vi "Add RPC Impl VIs.vi"(8 "error in":errorcluster, 9 "Application reference in":refnum<vi>, 10 "Service Impl class in":refnum<vi>, 11 "RPC Method Parameters":T1[](array[typedef])) -> (0 "error out":errorcluster, 3 "Service Impl class out":refnum<vi>)   [LabVIEW 2019, in "gRPC Template Creation Utility.lvlib"]
uses:
  gRPC Template Creation Utility.lvlib
  TypeDefs/RPC Method Parameters.ctl
  ServiceConstants.ctl
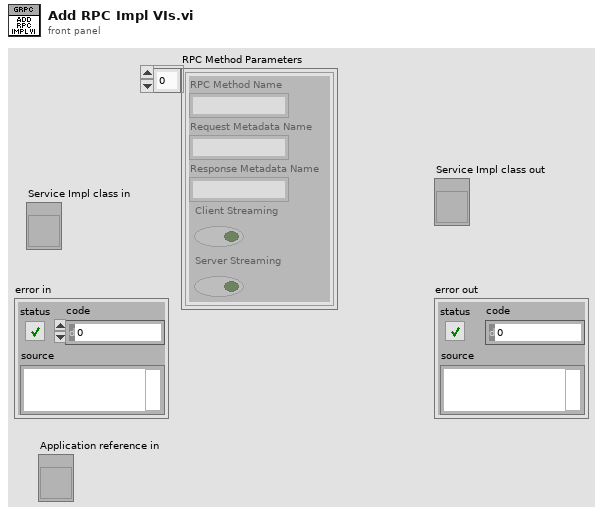
[diagram p1: front panel]
types:
  T1 = typedef "gRPC Template Creation Utility.lvlib/RPC Method Parameters.ctl" = cluster{"RPC Method Name":string, "Request Metadata Name":string, "Response Metadata Name":string, "Client Streaming":bool, "Server Streaming":bool}
  T2 = typedef "gRPC Template Creation Utility.lvlib/ServiceConstants.ctl" = enum16{"Stub", "Impl", "Usercode_server", "Generated_server", "RPC Service", "RPC Method package_service_method", "ServiceClass out", "ServiceClass in", "RPC Method"}
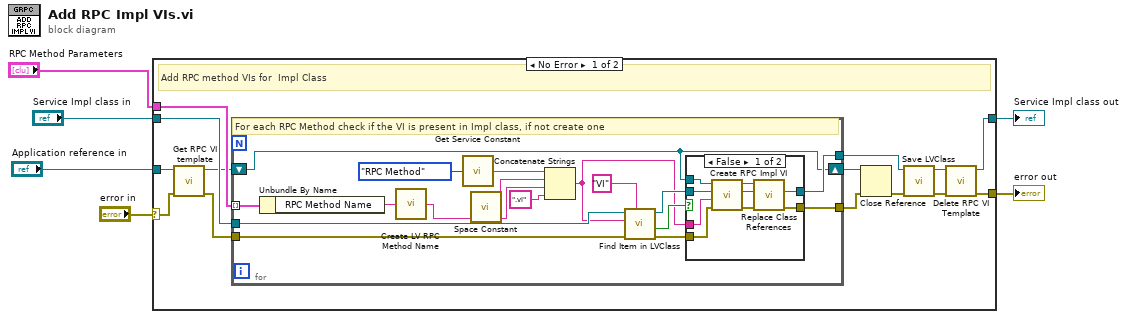
[diagram p0: block diagram]
diagram:
  n1 = case shown="No Error" "error in" {
    selector: "error in" -> [w15 w50]
    tunnel: [w20 w50] -> w5
    tunnel: "Service Impl class in" -> [w17 w49]
    tunnel: [w19 w49] -> w3
    tunnel: "RPC Method Parameters" -> [w18 _]
    tunnel: "Application reference in" -> [w16 _]
    frame No Error {
      # "Add RPC method VIs for  Impl Class"
      n2 = call "Get RPC VI template.vi"("error in (no error)"=w15, "Application in"=w16) -> ("error out"=w14:errorcluster, "Impl template RPC VI Reference"=w13:refnum<vi>)  [unwired: 7 in, 1 out]
      n3 = for {
        tunnel: w18 -> [w36] mode=indexing
        tunnel: w17 -> [w31]
        tunnel: w14 -> [w29]
        tunnel: [w27] -> w12
        tunnel: [w24] -> w10
        shift-right: [w23] -> w11
        shift-left: w13 -> [w23]
        # "For each RPC Method check if the VI is present in Impl class, if not create one"
        n4 = Unbundle By Name(w36) -> ("RPC Method Name"=w37:string)
        n5 = call "Create LV RPC Method Name.vi"("Proto Parser RPC Method Name in"=w37) -> ("LV RPC Method Name out"=w34:string)
        n6 = call "Get Service Constant.vi"("Service Constant Strings"=ServiceConstants."RPC Method") -> ("String Value"=w21:string)
        n7 = call <vilib>:"Space Constant.vi"() -> ("String"=w35:string)
        n8 = Concatenate Strings(w21, w35, w34, ".vi" ("string")) -> (w25:string)
        n9 = call "Find Item in LVClass.vi"("Item Type"="VI", "error in (no error)"=w29, "Item Name"=w25, "Class Item in"=w31) -> ("error out"=w28:errorcluster, "Found?"=w30:bool, "Class Item out"=w26:refnum<vi>)  [unwired: 4 in, 1 out]
        n10 = case shown="False" w30 {
          tunnel: w28 -> [w43 w48]
          tunnel: [w41 w48] -> w27
          tunnel: w26 -> [w42 w47]
          tunnel: w25 -> [w46 _]
          tunnel: [w38 w47] -> w24
          tunnel: w23 -> [w44 _]
          frame False {
            n11 = call "Create RPC Impl VI.vi"("error in (no error)"=w43, "String"=w46, "LVClassLibrary Item in"=w42, "Template VI in"=w44) -> ("error out"=w45:errorcluster, "LVClassLibrary out"=w40:refnum<vi>, "RPC Impl VI out"=w39:refnum<vi>)  [unwired: 5 in]
            n12 = call "Replace Class References.vi"("error in (no error)"=w45, "Target LVClassLibrary ref"=w40, "vi refnum"=w39) -> ("error out"=w41:errorcluster, "Target LVClassLibrary ref out"=w38:refnum<vi>)  [unwired: 7 in]
          }
          frame True {
          }
        }
      }
      n13 = Close Reference(reference=w11, error in (no error)=w12) -> (error out=w9:errorcluster)
      n14 = call "Save LVClass.vi"("error in (no error)"=w9, "LVClassLibrary in"=w10) -> ("error out"=w7:errorcluster, "LVClassLibrary out"=w8:refnum<vi>)  [unwired: 8 in]
      n15 = call "Delete RPC VI Template.vi"("error in (no error)"=w7, "LVClassLibrary in"=w8) -> ("error out"=w20:errorcluster, "LVClassLibrary out"=w19:refnum<vi>)  [unwired: 8 in]
    }
    frame Error {
    }
  }
  "error out" <- w5
  "Service Impl class out" <- w3
